vi "Class Adaptation Lesson 1.vi"() -> ()   [LabVIEW 2023]
doc: "Lesson 1 on the special adaptation that malleable VIs can do with LabVIEW classes."
uses:
  Cooling System/Cooling System.lvclass
  Thermal Sensor/Thermal Sensor.lvclass
  Thermal Test/Thermal Test.lvclass/Thermal Test.ctl
  Evaporative Cooler/Evaporative Cooler.lvclass
  J-Type Thermocouple/J-Type Thermocouple.lvclass
  5fe1d178-6f14-44e5-8d25-f9069cef54fd.vi
  918dc60a-d3f4-4a50-bca6-9040849fbea2.vi
  Thermal Test/Read Starting Temperature.vi
  Cooling System/Cool Until Target.vi
  Thermal Test/Run Test.vi
  Thermal Test/Check Result.vi
  Evaporative Cooler/Cool Until Target.vi
  J-Type Thermocouple/Read Temperature.vi
panel:
  out "pass? 2":bool[](array[boolean])
  out "pass? 1":bool[](array[boolean])
  # "Overview: This example assumes you are familiar with the basics of malleable VIs. In this example, you will learn how to use malleable VIs to define interfaces to allow the malleable VI to be reused on unrelated LabVIEW classes.\n\nIn LabVIEW 2017, a malleable VI that calls a method of class A accepts only data of class A or data of descendants of class A. \nIn later versions, the malleable VI also accepts data of other classes as long as the class has a public method with the same name and connector pane pattern as the method of class A that the malleable VI calls.\n\nYou can think of this as a form of dynamic dispatching but the dispatch is performed at edit time instead of run time. Because the dispatch is performed at edit time, classes passed to malleable VIs can reuse code without having to be related by inheritance. \n\nInstructions: \n1. Open the LabVIEW Class Hierarchy window. Notice that none of the classes in this example inherit from any of the other classes. This fact is important to understanding the example.\n2. Open the block diagram of this VI. Review the lessons presented there.\n3. Run the VI to see the pass/fail results. Each time you run, the data is randomly generated. This means that, by design, as part of this demo, most iterations will see some failures.\n4. Once you have finished reviewing this VI, open the Lesson 2 VI in the Malleable VIs - Class Adaptation example project."
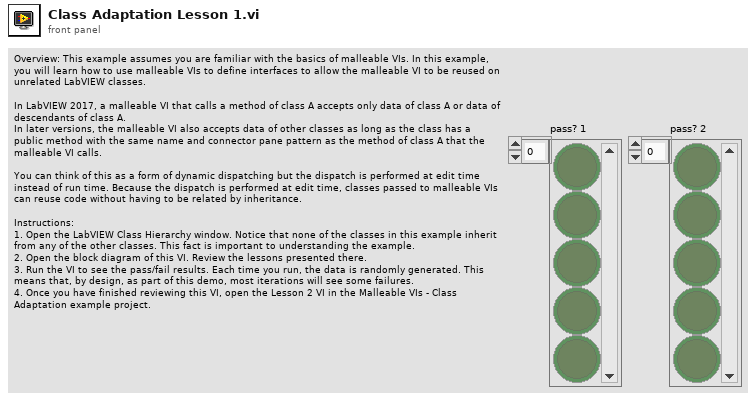
[diagram p1: front panel]
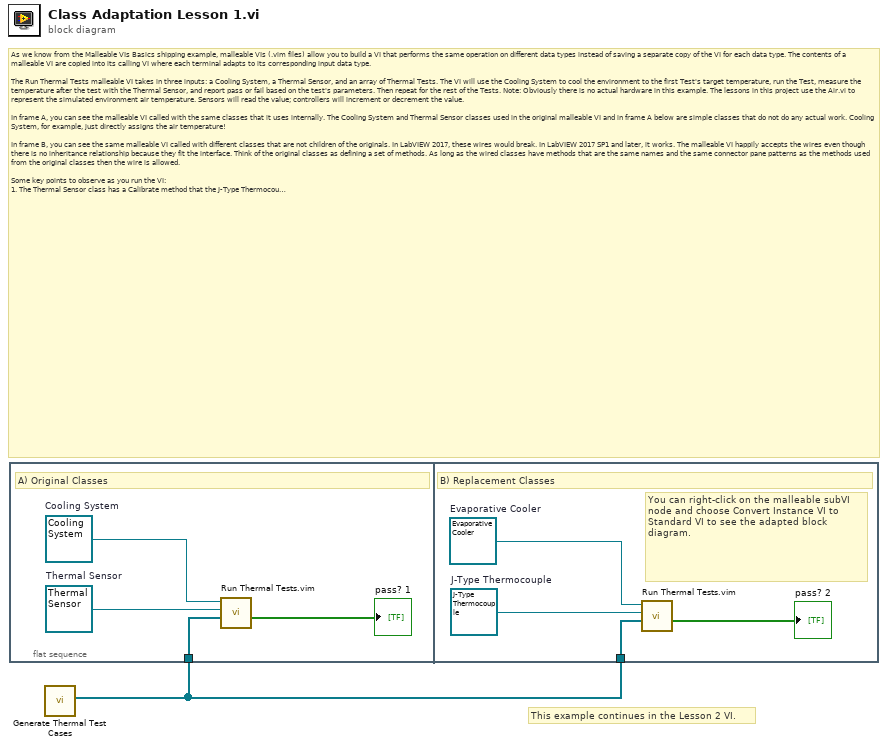
[diagram p0: block diagram]
diagram:
  # "This example continues in the Lesson 2 VI."
  # "As we know from the Malleable VIs Basics shipping example, malleable VIs (.vim files) allow you to build a VI that performs the same operation on different data types instead of saving a separate copy of the VI for each data type. The contents of a malleable VI are copied into its calling VI where each terminal adapts to its corresponding input data type.\n\nThe Run Thermal Tests malleable VI takes in three inputs: a Cooling System, a Thermal Sensor, and an array of Thermal Tests. The VI will use the Cooling System to cool the environment to the first Test's target temperature, run the Test, measure the temperature after the test with the Thermal Sensor, and report pass or fail based on the test's parameters. Then repeat for the rest of the Tests. Note: Obviously there is no actual hardware in this example. The lessons in this project use the Air.vi to represent the simulated environment air temperature. Sensors will read the value; controllers will increment or decrement the value.\n\nIn frame A, you can see the malleable VI called with the same classes that it uses internally. The Cooling System and Thermal Sensor classes used in the original malleable VI and in frame A below are simple classes that do not do any actual work. Cooling System, for example, just directly assigns the air temperature!\n\nIn frame B, you can see the same malleable VI called with different classes that are not children of the originals. In LabVIEW 2017, these wires would break. In LabVIEW 2017 SP1 and later, it works. The malleable VI happily accepts the wires even though there is no inheritance relationship because they fit the interface. Think of the original classes as defining a set of methods. As long as the wired classes have methods that are the same names and the same connector pane patterns as the methods used from the original classes then the wire is allowed. \n\nSome key points to observe as you run the VI: \n1. The Thermal Sensor class has a Calibrate method that the J-Type Thermocouple does not have. To use a malleable VI, the wired class must have all the methods used in the malleable VI but not all the methods of the original class. \n2. The Read Sensor method is dynamic dispatch in the original and static dispatch in the replacement. Dispatching differences are acceptable between the classes.\n3. The Evaporative Cooler has more methods than the original Cooling System class. It is acceptable to have more methods than are needed by the interface."
  n1 = flat-sequence {
    tunnel: w1 -> [w2]
    tunnel: w1 -> [w8]
    frame #0 {
      w4 = refnum<class "Thermal Sensor.lvclass"> refnum  # Thermal Sensor
      w5 = refnum<class "Cooling System.lvclass"> refnum  # Cooling System
      # "A) Original Classes"
      n2 = call "Run Thermal Tests.vim"("array of tests"=w2, "thermal sensor"=w4, "cooling system"=w5) -> ("pass?"=→"pass? 1":bool[])  [unwired: 7 in, 1 out]
    }
    frame #1 {
      w7 = refnum<class "J-Type Thermocouple.lvclass"> refnum  # J-Type Thermocouple
      w6 = refnum<class "Evaporative Cooler.lvclass"> refnum  # Evaporative Cooler
      # "You can right-click on the malleable subVI node and choose Convert Instance VI to Standard VI to see the adapted block diagram."
      # "B) Replacement Classes"
      n3 = call "Run Thermal Tests.vim"("array of tests"=w8, "thermal sensor"=w7, "cooling system"=w6) -> ("pass?"=→"pass? 2":bool[])  [unwired: 7 in, 1 out]
    }
  }
  n4 = call "Generate Thermal Test Cases.vi"() -> ("Array"=w1:refnum<class "Thermal Test.lvclass">[])  [unwired: 11 in]
